vi "cw_1_3.vi"() -> ()   [LabVIEW 2022 SP3]
panel:
  out "Seconds":i32
  out "Minutes":i32
  out "Hours":i32
  out "Days":i32
  out "Weeks":i32
  in  "Seconds":i32
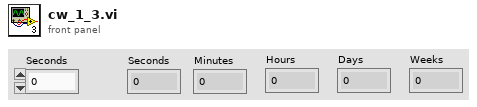
[diagram p1: front panel]
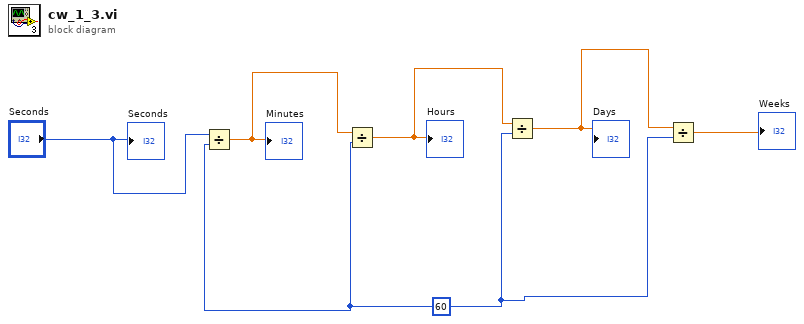
[diagram p0: block diagram]
diagram:
  w1 = 60
  n1 = Divide(x="Seconds", y=w1) -> (x/y=w5:dbl)
  "Minutes" <- w5
  n2 = Divide(x=w5, y=w1) -> (x/y=w4:dbl)
  "Hours" <- w4
  n3 = Divide(x=w4, y=w1) -> (x/y=w3:dbl)
  "Days" <- w3
  n4 = Divide(x=w3, y=w1) -> (x/y=→"Weeks":dbl)
  "Seconds" <- "Seconds"
